vi "Add Processor.vi"(8 "error in (no error)":errorcluster, 9 "Processor In":refnum<class "Image Processor.lvclass">, 10 "Label":string, 11 "ImagePipeline in":refnum<class "ImagePipeline.lvclass">) -> (0 "error out":errorcluster, 3 "ImagePipeline out":refnum<class "ImagePipeline.lvclass">)   [LabVIEW 2020, in "ImagePipeline.lvlib" / "ImagePipeline.lvclass"]
uses:
  ImagePipeline.lvclass
  C:/Program Files/National Instruments/LabVIEW 2020/vi.lib/ActorFramework/Actor/Actor.lvclass
  Image Processor/Image Processor/Image Processor.lvclass
  ImagePipeline.lvclass/ImagePipeline.ctl
  <vilib>/ActorFramework/Actor/Actor.lvclass
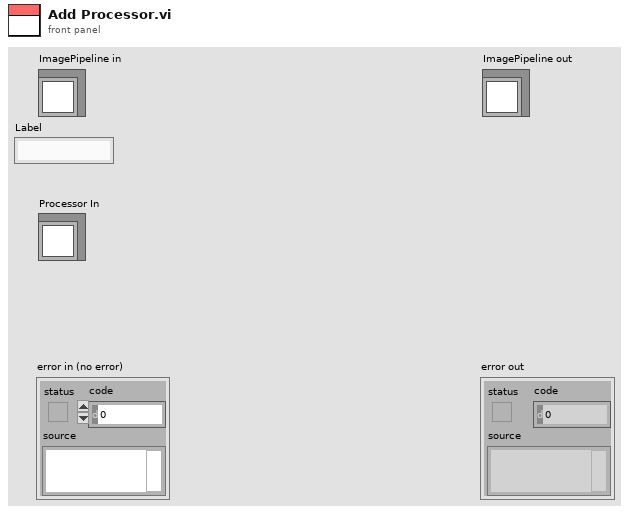
[diagram p1: front panel]
types:
  T1 = map{string, refnum<class "Message Enqueuer.lvclass">}
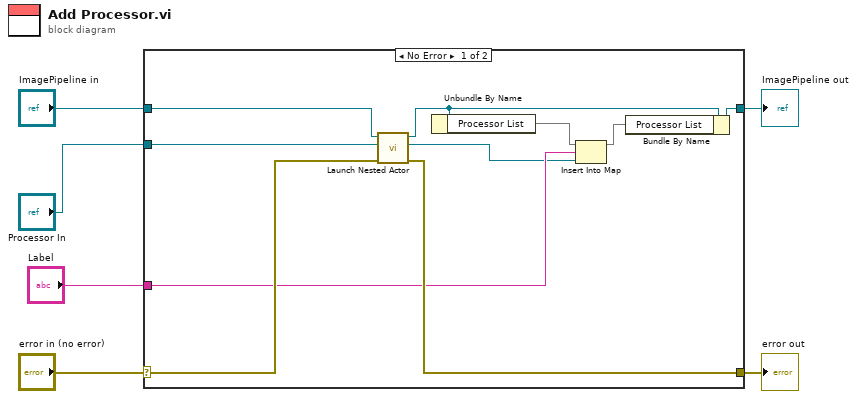
[diagram p0: block diagram]
diagram:
  n1 = case shown="No Error" "error in (no error)" {
    selector: "error in (no error)" -> [w15 w18]
    tunnel: [w14 w18] -> w5
    tunnel: [w12 w17] -> w3
    tunnel: "ImagePipeline in" -> [w16 w17]
    tunnel: "Processor In" -> [w13 _]
    tunnel: "Label" -> [w9 _]
    frame No Error {
      n2 = call <vilib>:"Launch Nested Actor.vi"("error in (no error)"=w15, "Nested Actor"=w13, "Caller Actor in"=w16) -> ("error out"=w14:errorcluster, "Nested Actor's Enqueuer"=w8:refnum<class "Message Enqueuer.lvclass">, "Caller Actor out"=w11:refnum<class "ImagePipeline.lvclass">)  [unwired: 6 in]
      n3 = Unbundle By Name(w11) -> ("Processor List"=w10:T1)
      n4 = Insert Into Map(map in=w10, key=w9, value=w8) -> (map out=w7:T1)  [unwired: 2 out]
      n5 = Bundle By Name(cluster=w11, "Processor List"=w7) -> (w12:refnum<class "ImagePipeline.lvclass">)
    }
    frame Error {
    }
  }
  "error out" <- w5
  "ImagePipeline out" <- w3
